vi "Vision Calculations.vi"(0 "Image In":T2, 3 "error in":errorcluster) -> (5 "Vision Data":T1)   [LabVIEW 2013]
uses:
  <vilib>/vision/Image Controls.llb/IMAQ Image.ctl
  typedefs/vision data.ctl
  <vilib>/vision/NI_Vision_Development_Module.lvlib
panel:
  out "Aspect\nScore":dbl
  out "Rect Score":dbl
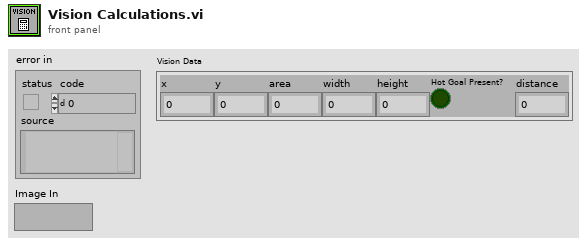
[diagram p1: front panel]
types:
  T1 = typedef "vision data.ctl" = cluster{"x":dbl, "y":dbl, "area":dbl, "width":dbl, "height":dbl, "Hot Goal Present?":bool, "distance":dbl}
  T2 = typedef "IMAQ Image.ctl" = refnum<image>
  T3 = typedef "Particle Parameters" = i32
  T4 = cluster{"Area":dbl, "Number of Holes":dbl, "Bounding Rect":cluster{"Left":dbl, "Top":dbl, "Right":dbl, "Bottom":dbl}, "Center of Mass":cluster{"X":dbl, "Y":dbl}, "Orientation":dbl, "Dimensions":cluster{"Width":dbl, "Height":dbl}}[]
  T5 = cluster{"Horizontal":bool, "Aspect Score":dbl, "Rect Score":dbl, "Rectangle":cluster{"Left":dbl, "Top":dbl, "Right":dbl, "Bottom":dbl}, "Equiv H":dbl, "Equiv V":dbl}
  T6 = cluster{"Area":dbl, "Number of Holes":dbl, "Bounding Rect":cluster{"Left":dbl, "Top":dbl, "Right":dbl, "Bottom":dbl}, "Center of Mass":cluster{"X":dbl, "Y":dbl}, "Orientation":dbl, "Dimensions":cluster{"Width":dbl, "Height":dbl}}
  T7 = cluster{"Left":dbl, "Top":dbl, "Right":dbl, "Bottom":dbl}
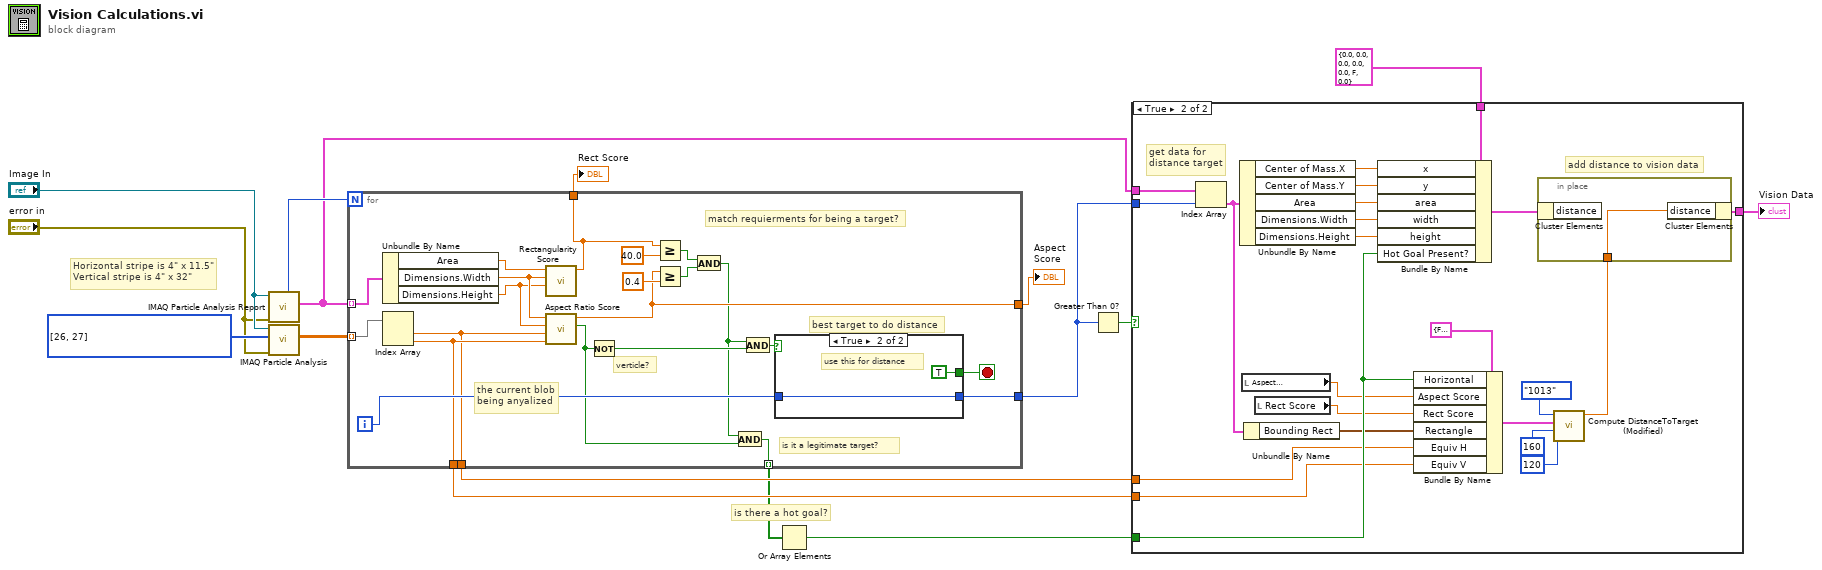
[diagram p0: block diagram]
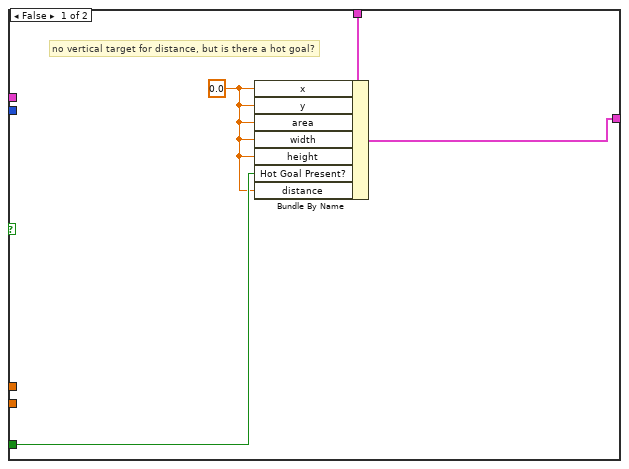
[diagram p2: hidden frame]
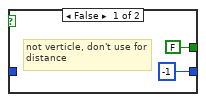
[diagram p3: hidden frame]
diagram:
  w14 = T3[] [26, 27] items=["Center of Mass X", "Center of Mass Y", "First Pixel X", "First Pixel Y", "Bounding Rect Left", "Bounding Rect Top", "Bounding Rect Right", "Bounding Rect Bottom", "Max Feret Diameter Start X", "Max Feret Diameter Start Y", "Max Feret Diameter End X", "Max Feret Diameter End Y", "Max Horiz. Segment Length Left", "Max Horiz. Segment Length Right", "Max Horiz. Segment Length Row", "-", "Bounding Rect Width", "Bounding Rect Height", "Bounding Rect Diagonal", "Perimeter", "Convex Hull Perimeter", "Holes' Perimeter", "Max Feret Diameter", "Equivalent Ellipse Major Axis", "Equivalent Ellipse Minor Axis", "Equivalent Ellipse Minor Axis (Feret)", "Equivalent Rect Long Side", "Equivalent Rect Short Side", "Equivalent Rect Diagonal", "Equivalent Rect Short Side (Feret)", "Average Horiz. Segment Length", "Average Vert. Segment Length", "Hydraulic Radius", "Waddel Disk Diameter", "-", "Area", "Holes' Area", "Particle & Holes' Area", "Convex Hull Area", "Image Area", "-", "Number of Holes", "Number of Horiz. Segments", "Number of Vert. Segments", "-", "Orientation", "Max Feret Diameter Orientation", "-", "% Area/Image Area", "% Area/(Particle & Holes' Area)", "Ratio of Equivalent Ellipse Axes", "Ratio of Equivalent Rect Sides", "-", "Elongation Factor", "Compactness Factor", "Heywood Circularity Factor", "Type Factor", "-", "Sum X", "Sum Y", "Sum XX", "Sum XY", "Sum YY", "Sum XXX", "Sum XXY", "Sum XYY", "Sum YYY", "-", "Moment of Inertia XX", "Moment of Inertia XY", "Moment of Inertia YY", "Moment of Inertia XXX", "Moment of Inertia XXY", "Moment of Inertia XYY", "Moment of Inertia YYY", "Norm. Moment of Inertia XX", "Norm. Moment of Inertia XY", "Norm. Moment of Inertia YY", "Norm. Moment of Inertia XXX", "Norm. Moment of Inertia XXY", "Norm. Moment of Inertia XYY", "Norm. Moment of Inertia YYY", "Hu Moment 1", "Hu Moment 2", "Hu Moment 3", "Hu Moment 4", "Hu Moment 5", "Hu Moment 6", "Hu Moment 7"] ("Pixel Measurements")
  # "Horizontal stripe is 4\" x 11.5\"\nVertical stripe is 4\" x 32\""
  # "is there a hot goal?"
  n1 = call "IMAQ Particle Analysis Report"("error in (no error)"="error in", "Image"="Image In") -> ("Particle Reports (Pixels)"=w11:T4, "Number of Particles"=w16:i32)  [unwired: 4 in, 4 out]
  n2 = call "IMAQ Particle Analysis"("error in (no error)"="error in", "Pixel Measurements"=w14, "Image"="Image In") -> ("Particle Measurements (Pixels)"=w13:dbl[][])  [unwired: 3 in, 5 out]
  n3 = for {
    N: w16 -> [_]
    tunnel: w11 -> [w37] mode=indexing
    tunnel: w13 -> [w36] mode=indexing
    tunnel: [w26] -> w4
    tunnel: [w23] -> w9
    tunnel: [w22] -> w8
    tunnel: [w21] -> w6
    tunnel: [w20] -> w7
    tunnel: [w17] -> w1 mode=indexing
    i -> [w25]
    stop <- w32 stop-if-true
    # "is it a legitimate target?"
    # "the current blob\nbeing anyalized"
    # "match requierments for being a target?"
    # "best target to do distance"
    # "verticle?"
    n4 = Unbundle By Name(w37) -> ("Area"=w35:dbl, "Dimensions.Width"=w34:dbl, "Dimensions.Height"=w33:dbl)
    n5 = Index Array(array=w36) -> (element #1=w20:dbl, element #2=w21:dbl)  [unwired: 2 in]
    n6 = call "Rectangularity Score.vi"("Height"=w33, "Width"=w34, "Area"=w35) -> ("Score"=w23:dbl)  [unwired: 8 in]
    n7 = call "Aspect Ratio Score.vi"("Equivalent Rect Short"=w21, "Equivalent Rect Long"=w20, "Height"=w33, "Width"=w34) -> ("Horizontal"=w18:bool, "Score"=w22:dbl)  [unwired: 6 in]
    n8 = Not(x=w18) -> (.not. x?=w24:bool)
    n9 = Greater Or Equal?(x=w23, y=40.0) -> (x >= y?=w28:bool)
    n10 = Greater Or Equal?(x=w22, y=0.4) -> (x >= y?=w29:bool)
    n11 = And(x=w28, y=w29) -> (x .and. y?=w19:bool)
    n12 = And(x=w19, y=w18) -> (x .and. y?=w17:bool)
    n13 = And(x=w19, y=w24) -> (x .and. y?=w27:bool)
    n14 = case shown="True" w27 {
      tunnel: w25 -> [_ w41]
      tunnel: [-1 w41] -> w26
      tunnel: [FALSE TRUE] -> w32
      frame False {
        # "not verticle, don't use for\ndistance"
      }
      frame True {
        # "use this for distance"
      }
    }
  }
  "Rect Score" <- w9
  "Aspect\nScore" <- w8
  n15 = Or Array Elements(Boolean array=w1) -> (logical OR=w10:bool)
  n16 = Greater Than 0?(x=w4) -> (x > 0?=w3:bool)
  n17 = case shown="True" w3 {
    tunnel: w11 -> [_ w68]
    tunnel: w10 -> [w43 w60]
    tunnel: w7 -> [_ w55]
    tunnel: w6 -> [_ w54]
    tunnel: [w44 w49] -> w5
    tunnel: w4 -> [_ w47]
    tunnel: T1 {"x"=0.0, "y"=0.0, "area"=0.0, "width"=0.0, "height"=0.0, "Hot Goal Present?"=FALSE, "distance"=0.0} ("Data") -> [w45 w46]
    frame False {
      w42 = 0.0
      # "no vertical target for distance, but is there a hot goal?"
      n18 = Bundle By Name(cluster=w45, "x"=w42, "y"=w42, "area"=w42, "width"=w42, "height"=w42, "Hot Goal Present?"=w43, "distance"=w42) -> (w44:T1)
    }
    frame True {
      # "add distance to vision data"
      # "get data for \ndistance target"
      n19 = Index Array(array=w68, index=w47) -> (element=w59:T6)
      n20 = Unbundle By Name(w59) -> ("Center of Mass.X"=w67:dbl, "Center of Mass.Y"=w66:dbl, "Area"=w65:dbl, "Dimensions.Width"=w64:dbl, "Dimensions.Height"=w63:dbl)
      n21 = local read "Aspect\nScore"() -> (w56:dbl)
      n22 = Unbundle By Name(w59) -> ("Bounding Rect"=w58:T7)
      n23 = local read "Rect Score"() -> (w57:dbl)
      n24 = Bundle By Name(cluster=w46, "x"=w67, "y"=w66, "area"=w65, "width"=w64, "height"=w63, "Hot Goal Present?"=w60) -> (w50:T1)
      n25 = Bundle By Name(cluster=T5 {"Horizontal"=FALSE, "Aspect Score"=0.0, "Rect Score"=0.0, "Rectangle"={"Left"=0.0, "Top"=0.0, "Right"=0.0, "Bottom"=0.0}, "Equiv H"=0.0, "Equiv V"=0.0} ("Vertical Strip"), "Horizontal"=w60, "Aspect Score"=w56, "Rect Score"=w57, "Rectangle"=w58, "Equiv H"=w55, "Equiv V"=w54) -> (w61:T5)
      n26 = call "Compute DistanceToTarget (Modified).vi"("Y Image Resolution"=120, "X Image Resolution"=160, "Vertical Strip"=w61, "Camera Type"=enum16{"206", "1011", "1013"}."1013") -> ("Distance to Goal Wall (ft)"=w48:dbl)  [unwired: 5 in, 2 out]
      n27 = in-place {
        in-place-border: w48 -> [w69]
        n28 = in-place-cluster #1(w50) -> ()  [unwired: 1 out]
        n29 = in-place-cluster #1("distance"=w69) -> (w49:T1)
      }
    }
  }
  "Vision Data" <- w5
